vi "Write Header.vi"(6 "Metadata":variant, 8 "error in (no error)":errorcluster, 11 "CubeLogger in":refnum<class "CubeLogger.lvclass">) -> (0 "error out":errorcluster, 2 "Canceled?":bool, 3 "CubeLogger out":refnum<class "CubeLogger.lvclass">)   [LabVIEW 2018, in "CubeLogger.lvclass"]
uses:
  CubeLogger.lvclass
  Dataset.ctl
  CubeLogger.lvclass/CubeLogger.ctl
  <vilib>/addons/_JKI.lib/Serialization/JSON/JKI JSON Serialization.lvlib
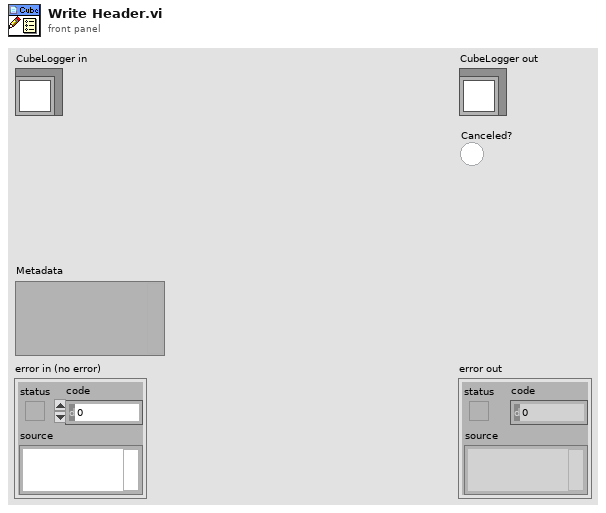
[diagram p1: front panel]
types:
  T1 = typedef "CubeLogger.lvclass/Dataset.ctl" = cluster{"name":string, "path":string, "size":i32[], "type":enum16{"single", "double", "uint8", "uint16", "uint32", "uint64", "int8", "int16", "int32", "int64"}, "mfmt":string}
  T2 = cluster{"name":string, "desc":string, "data":string, "meta":string}
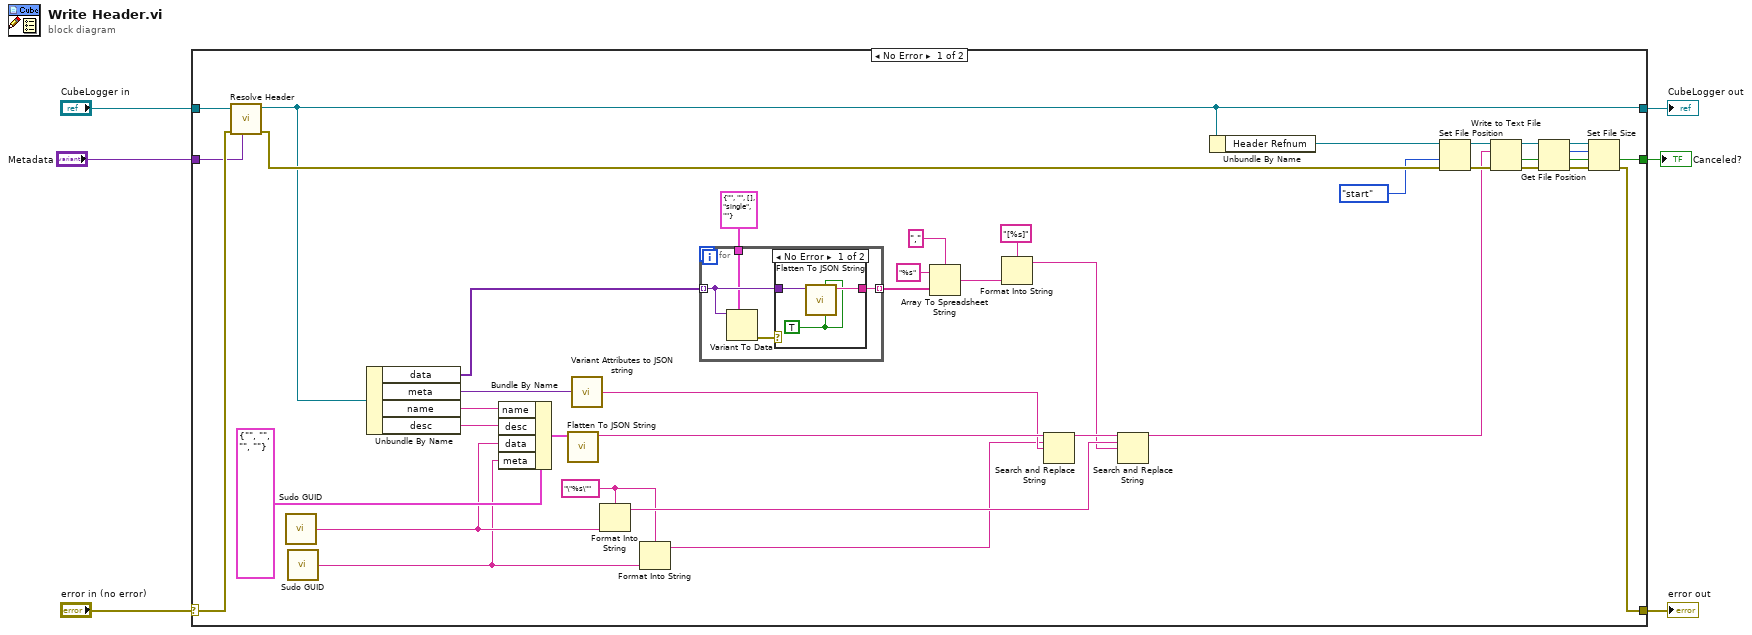
[diagram p0: block diagram]
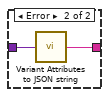
[diagram p2: hidden frame]
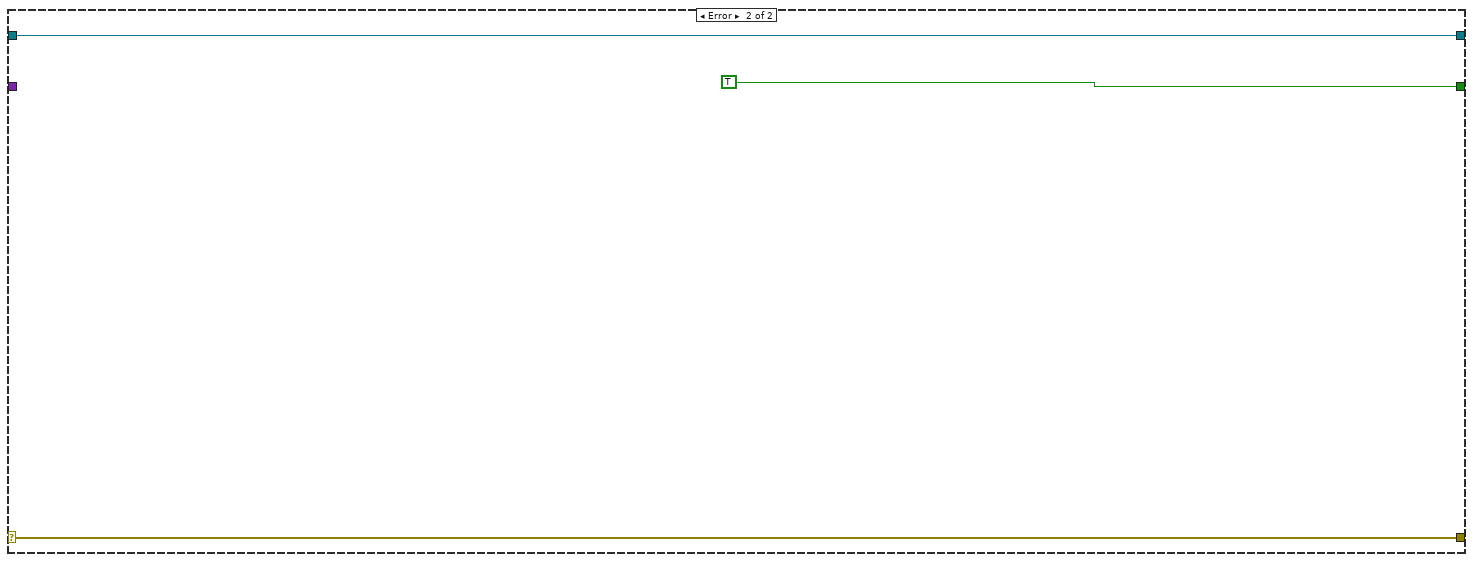
[diagram p3: hidden frame]
diagram:
  n1 = case shown="No Error" "error in (no error)" {
    selector: "error in (no error)" -> [w42 w55]
    tunnel: [w7 w55] -> w5
    tunnel: [w19 w54] -> w3
    tunnel: "CubeLogger in" -> [w43 w54]
    tunnel: [w17 TRUE] -> w2
    tunnel: "Metadata" -> [w16 _]
    frame No Error {
      w29 = "\"%s\"" ("format string")
      n2 = call-dynamic "Resolve Header.vi"("Metadata"=w16, "error in (no error)"=w42, "CubeLogger in"=w43) -> ("error out"=w20:errorcluster, "CubeLogger out"=w19:refnum<class "CubeLogger.lvclass">)  [unwired: 7 in]
      n3 = call "Sudo GUID.vi"() -> ("GUID String"=w32:string)  [unwired: 5 in]
      n4 = call "Sudo GUID.vi"() -> ("GUID String"=w31:string)  [unwired: 5 in]
      n5 = Unbundle By Name(w19) -> ("data"=w28:variant[], "meta"=w37:variant, "name"=w40:string, "desc"=w39:string)
      n6 = Bundle By Name(cluster=T2 {"name"="", "desc"="", "data"="", "meta"=""} ("Header"), "name"=w40, "desc"=w39, "data"=w32, "meta"=w31) -> (w38:T2)
      n7 = call <vilib>:"Flatten To JSON String.vi"("Variant"=w38) -> ("JSON String"=w36:string)  [unwired: 9 in, 1 out]
      n8 = call "Variant Attributes to JSON string.vi"("Variant Attributes"=w37) -> ("String"=w35:string)
      n9 = Format Into String(format string=w29, w32) -> (resulting string=w33:string)  [unwired: 2 in, 1 out]
      n10 = Format Into String(format string=w29, w31) -> (resulting string=w30:string)  [unwired: 2 in, 1 out]
      n11 = for {
        tunnel: w28 -> [w45] mode=indexing
        tunnel: [w46] -> w24 mode=indexing
        tunnel: T1 {"name"="", "path"="", "size"=[], "type"=enum."single", "mfmt"=""} ("CubeLogger.lvclass:Dataset") -> [w44]
        n12 = Variant To Data(type=w44, Variant=w45) -> (error out=w47:errorcluster)  [unwired: 1 in, 1 out]
        n13 = case shown="No Error" w47 {
          tunnel: [w50 w51] -> w46
          tunnel: w45 -> [w49 w52]
          frame No Error {
            w48 = TRUE ("Enums As String (F)")
            n14 = call <vilib>:"Flatten To JSON String.vi"("Enums As String (F)"=w48, "Numeric Extensions (F)"=w48, "Variant"=w49) -> ("JSON String"=w50:string)  [unwired: 7 in, 1 out]
          }
          frame Error {
            n15 = call "Variant Attributes to JSON string.vi"("Variant Attributes"=w52) -> ("String"=w51:string)
          }
        }
      }
      n16 = Array To Spreadsheet String(delimiter (Tab)=",", array=w24, 3:"%s" ("format string")) -> (spreadsheet string=w23:string)
      n17 = Format Into String(format string="[%s]", w23) -> (resulting string=w21:string)  [unwired: 2 in, 1 out]
      n18 = Search and Replace String(input string=w36, search string=w30, replace string=w35) -> (result string=w34:string)  [unwired: 5 in, 3 out]
      n19 = Search and Replace String(input string=w34, search string=w33, replace string=w21) -> (result string=w18:string)  [unwired: 5 in, 3 out]
      n20 = Unbundle By Name(w19) -> ("Header Refnum"=w15:refnum<file>)
      n21 = Set File Position(refnum=w15, from (0:start)=enum16{"start", "end", "current"}."start") -> (refnum out=w14:refnum<file>)  [unwired: 2 in, 1 out]
      n22 = Write to Text File(file (use dialog)=w14, text=w18, error in=w20) -> (refnum out=w11:refnum<file>, cancelled=w17:bool, error out=w12:errorcluster)  [unwired: 1 in]
      n23 = Get File Position(4:w12, 7:w11) -> (0:w10:errorcluster, 2:w9:i64, 3:w8:refnum<file>)
      n24 = Set File Size(4:w10, 6:w9, 7:w8) -> (0:w7:errorcluster)  [unwired: 1 out]
    }
    frame Error {
    }
  }
  "error out" <- w5
  "CubeLogger out" <- w3
  "Canceled?" <- w2
